vi "test Hybrid DIO.vi"(8 "error in (no error)":errorcluster, 11 "TestCase in":refnum<class "cRIO System Tests.lvclass">) -> (0 "error out":errorcluster, 3 "TestCase out":refnum<class "cRIO System Tests.lvclass">)   [LabVIEW 2019, in "cRIO System Tests.lvclass"]
uses:
  cRIO System Tests.lvclass
  C:/Users/nitest/Desktop/Git 2019/niveristand-custom-device-testing-tools/VeriStandTestCase/VeriStandTestCase.lvclass
  <vilib>/numeric/sub_Random U32.vi
  <vilib>/numeric/Random Number (Range) U64.vi
  <vilib>/addons/_JKI Toolkits/VI Tester/TestCase.llb/TestCase.lvclass
  niveristand-custom-device-testing-tools/VeriStandTestCase/VeriStandTestCase.lvclass
  C:/Program Files (x86)/National Instruments/LabVIEW 2019/vi.lib/addons/_JKI Toolkits/VI Tester/TestCase.llb/TestCase.lvclass
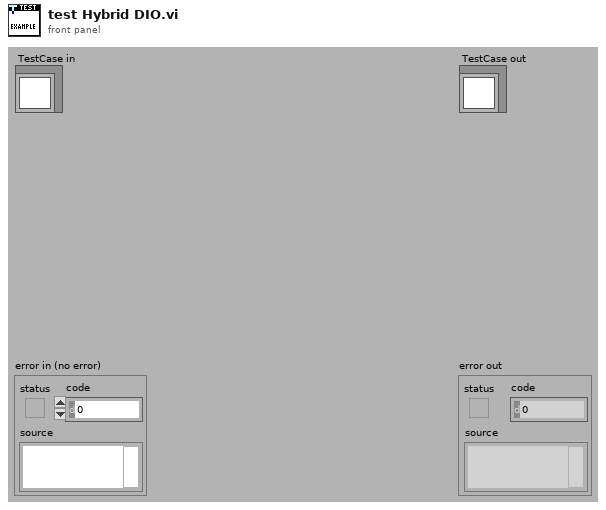
[diagram p1: front panel]
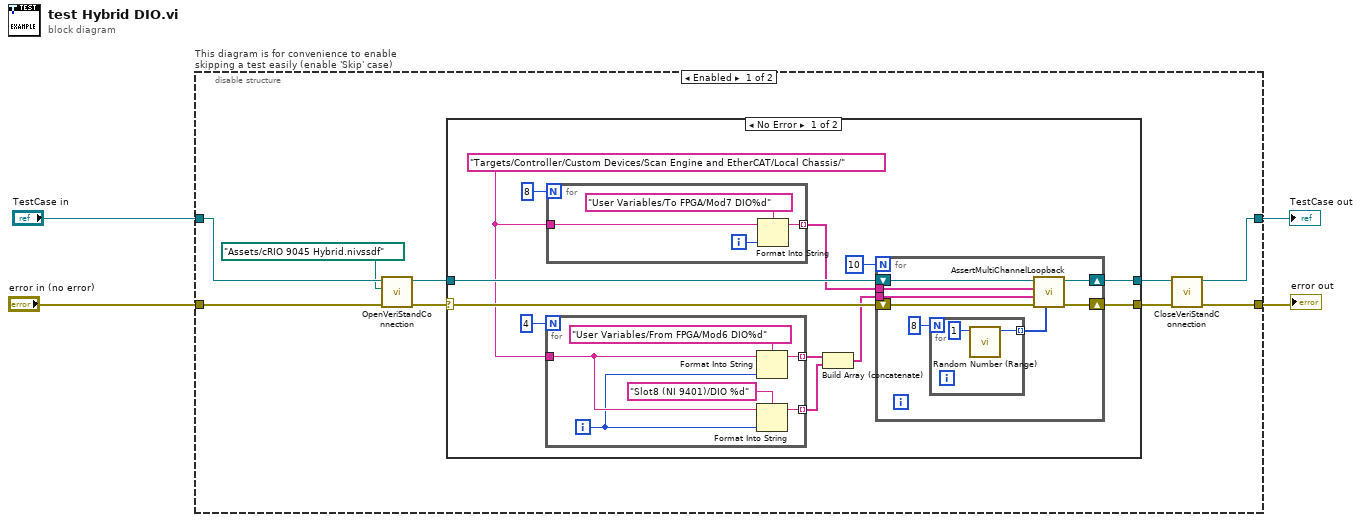
[diagram p0: block diagram]
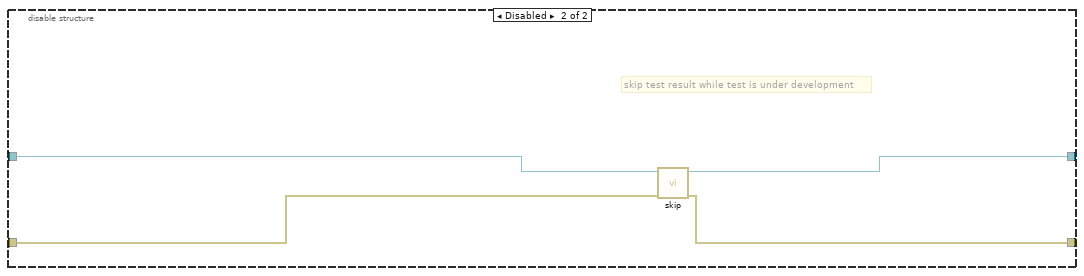
[diagram p3: hidden frame]
diagram:
  n1 = disable-structure "This diagram is for convenience to enable skipping a test easily (enable 'Skip' case)" shown="Enabled" {
    disable-tunnel: "TestCase in" -> [w10 w51]
    disable-tunnel: [w6 w49] -> w1
    disable-tunnel: [w8 w50] -> w3
    disable-tunnel: "error in (no error)" -> [w12 w48]
    frame Enabled {
      n2 = call-dynamic "OpenVeriStandConnection.vi"("error in (no error)"=w12, "System Definition File"=path "Assets/cRIO 9045 Hybrid.nivssdf", "VeriStand Test Case in"=w10) -> ("error out"=w13:errorcluster, "VeriStand Test Case out"=w11:refnum<class "cRIO System Tests.lvclass">)  [unwired: 6 in, 1 out]
      n3 = case shown="No Error" w13 {
        selector: w13 -> [w22 w47]
        tunnel: [w21 w47] -> w9
        tunnel: [w23 w46] -> w7
        tunnel: w11 -> [w24 w46]
        frame No Error {
          w14 = "Targets/Controller/Custom Devices/Scan Engine and EtherCAT/Local Chassis/"
          n4 = for {
            N: 4 -> [_]
            tunnel: w14 -> [w33]
            tunnel: [w34] -> w17 mode=indexing
            tunnel: [w31] -> w16 mode=indexing
            i -> [w30]
            n5 = Format Into String(format string="User Variables/From FPGA/Mod6 DIO%d", initial string=w33, w30) -> (resulting string=w34:string)  [unwired: 1 in, 1 out]
            n6 = Format Into String(format string="Slot8 (NI 9401)/DIO %d", initial string=w33, w30) -> (resulting string=w31:string)  [unwired: 1 in, 1 out]
          }
          n7 = for {
            N: 8 -> [_]
            tunnel: w14 -> [w26]
            tunnel: [w28] -> w20 mode=indexing
            i -> [w27]
            n8 = Format Into String(format string="User Variables/To FPGA/Mod7 DIO%d", initial string=w26, w27) -> (resulting string=w28:string)  [unwired: 1 in, 1 out]
          }
          n9 = Build Array (concatenate)(w17, w16) -> (w15:string[])
          n10 = for {
            N: 10 -> [_]
            tunnel: w20 -> [w39]
            tunnel: w15 -> [w38]
            shift-right: [w42] -> w23
            shift-left: w24 -> [w43]
            shift-right: [w40] -> w21
            shift-left: w22 -> [w41]
            n11 = for {
              N: 8 -> [_]
              tunnel: [w45] -> w36 mode=indexing
              n12 = call-poly <vilib>:"Random Number (Range).vi"("upper bound (100)"=u64 1) -> ("number"=w45:u64)  [unwired: 10 in]
            }
            n13 = call "AssertMultiChannelLoopback.vi"("Values"=w36, "error in (no error)"=w41, "Read Channels"=w38, "Write Channels"=w39, "VeriStand Test Case in"=w43) -> ("error out"=w40:errorcluster, "VeriStand Test Case out"=w42:refnum<class "cRIO System Tests.lvclass">)  [unwired: 5 in]
          }
        }
        frame Error {
        }
      }
      n14 = call-dynamic "CloseVeriStandConnection.vi"("error in (no error)"=w9, "VeriStand Test Case in"=w7) -> ("error out"=w8:errorcluster, "VeriStand Test Case out"=w6:refnum<class "cRIO System Tests.lvclass">)  [unwired: 8 in]
    }
    frame Disabled {
      # "skip test result while test is under development"
      n15 = call <vilib>:"skip.vi"("error in (no error)"=w48, "TestCase in"=w51) -> ("error out"=w50:errorcluster, "TestCase out"=w49:refnum<class "cRIO System Tests.lvclass">)  [unwired: 8 in]
    }
  }
  "error out" <- w3
  "TestCase out" <- w1
